vi "FILE_DIALOG 2016.vi"(0 "flow_slope_IN":dbl=51.35 format="%.2f", 1 "pressure_slope_IN":dbl=23.33 format="%.2f", 3 "string_pot_slope_IN":dbl=1.5 format="%.2f", 4 "Descriptions":string[](array[string]), 5 "error in (no error)":errorcluster, 6 "start path":path=path "D:/Cascade/Data/Output Files", 7 "Sensor Cluster":T1, 10 "Array in":refnum<k24>[](array[refnum])) -> (8 "path":path, 9 "Sensor Cluster 2":T1, 11 "exists":bool, 12 "Array out":refnum<k24>[](array[refnum]), 14 "flow_slope_OUT":dbl=51.35 format="%.2f", 15 "pressure_slope_OUT":dbl=732.5347533511234 format="%.2f", 17 "string_pot_slope_OUT":dbl=1.5 format="%.2f", 19 "error out":errorcluster)   [LabVIEW 2016]
uses:
  C:/Program Files (x86)/National Instruments/LabVIEW 2016/vi.lib/ULx/ULx_LV.dll
  Program Files (x86)/National Instruments/LabVIEW 2016/vi.lib/ULx/ULx_LV.dll
  controls/MCC DAQ Readings.ctl
panel:
  out "Loop Counter":i32
  out "cal_completed":bool
  out "new_or _prev_file_selected":bool
  in  "calibrate_KPRO":bool
  in  "previous_file":bool
  in  "new_file":bool
  in  "OK Button":bool
  # "Select root file\nsuch as test.csv"
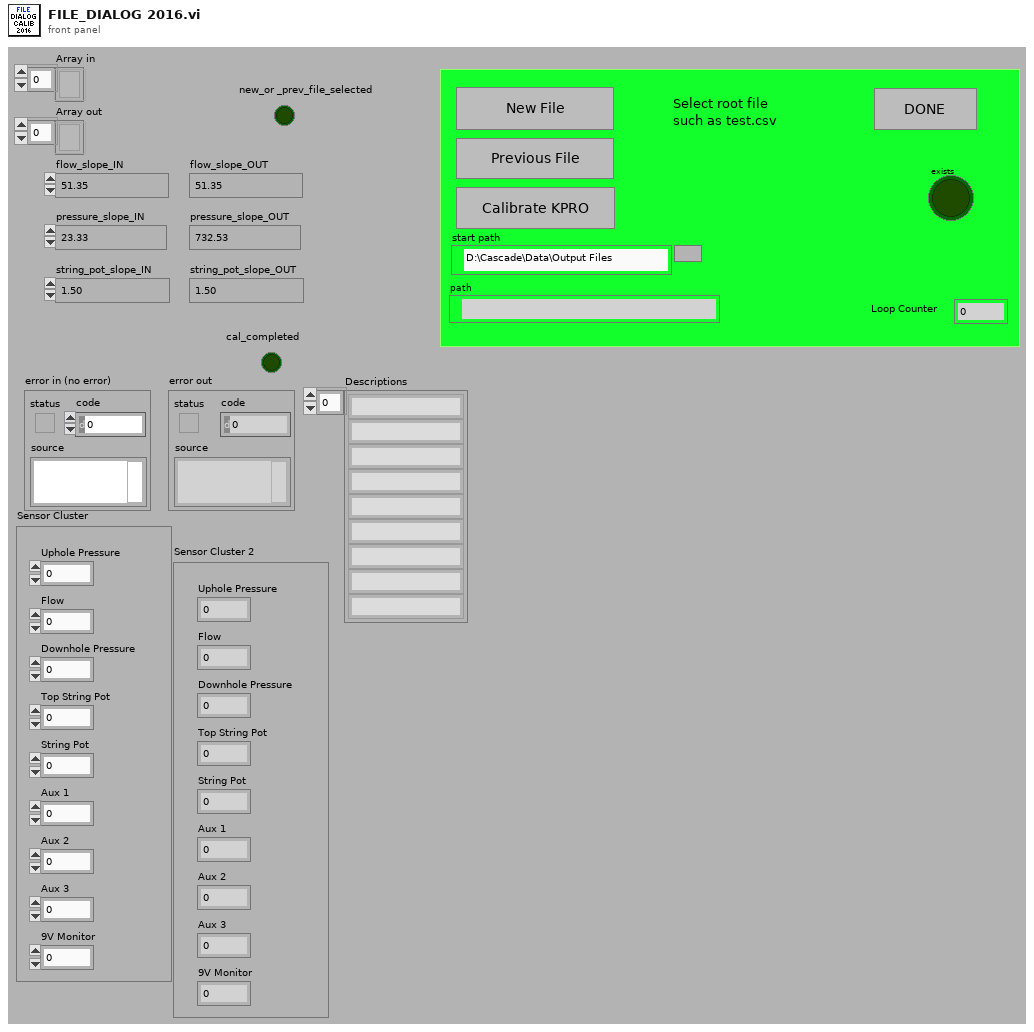
[diagram p1: front panel]
types:
  T1 = typedef "MCC DAQ Readings.ctl" = cluster{"Uphole Pressure":dbl, "Flow":dbl, "Downhole Pressure":dbl, "Top String Pot":dbl, "String Pot":dbl, "Aux 1":dbl, "Aux 2":dbl, "Aux 3":dbl, "9V Monitor":dbl}
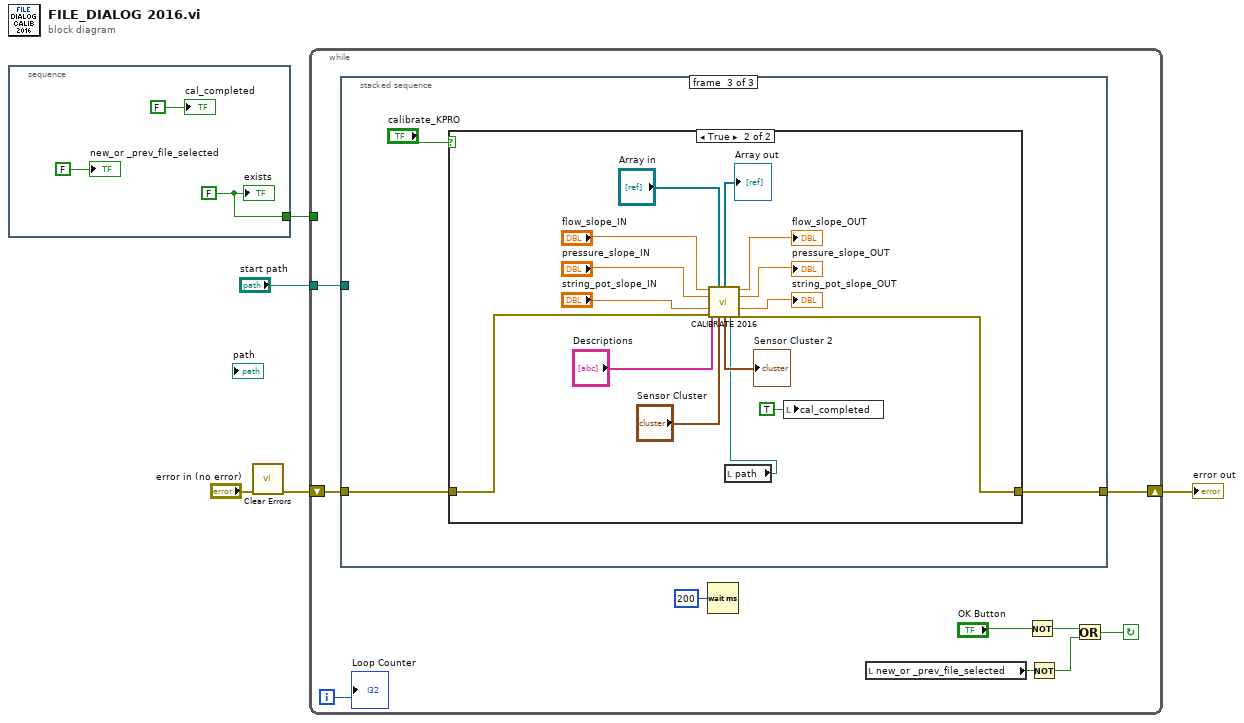
[diagram p0: block diagram]
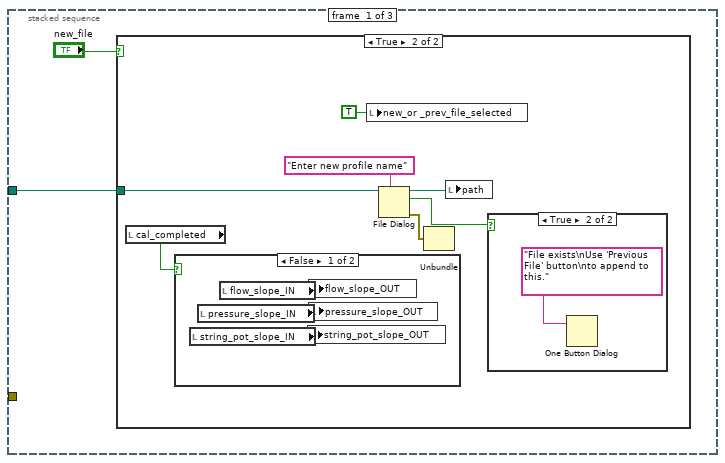
[diagram p2: hidden frame]
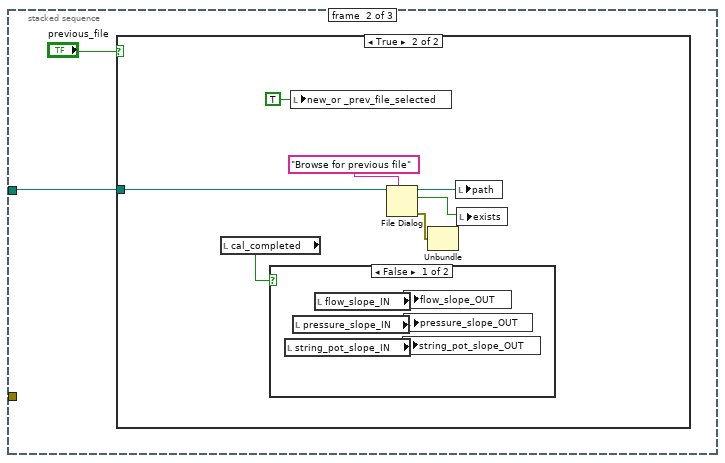
[diagram p6: hidden frame]
diagram:
  n1 = stacked-sequence {
    tunnel: [w8] -> w5
    frame #0 {
      w8 = FALSE ("exists")
      "exists" <- w8
      "new_or _prev_file_selected" <- FALSE ("new_or _prev_file_selected")
      "cal_completed" <- FALSE ("cal_completed")
    }
  }
  n2 = call <vilib>:"Clear Errors.vi"("error in (no error)"="error in (no error)") -> ("error out"=w1:errorcluster)  [unwired: 5 in, 1 out]
  n3 = while {
    shift-left: w1 -> [w15]
    shift-right: [w14] -> w2
    tunnel: "start path" -> [w16]
    tunnel: w5 -> [_]
    i -> [w9]
    stop <- w13 continue-if-true
    n4 = stacked-sequence {
      tunnel: w16 -> [w19 w32 _]
      tunnel: w15 -> [_ _ w45]
      tunnel: [_ _ w44] -> w14
      frame #0 {
        n5 = case shown="True" "new_file" {
          tunnel: w19 -> [_ w24]
          frame False {
          }
          frame True {
            n6 = local read "cal_completed"() -> (w22:bool)
            n7 = case shown="False" w22 {
              frame False {
                n8 = local read "string_pot_slope_IN"() -> (w28:dbl)
                n9 = local read "pressure_slope_IN"() -> (w29:dbl)
                n10 = local read "flow_slope_IN"() -> (w30:dbl)
                n11 = local write "string_pot_slope_OUT"(w28) -> ()
                n12 = local write "flow_slope_OUT"(w30) -> ()
                n13 = local write "pressure_slope_OUT"(w29) -> ()
              }
              frame True {
              }
            }
            n14 = local write "new_or _prev_file_selected"(TRUE ("new_or _prev_file_selected")) -> ()
            n15 = File Dialog(7:"Enter new profile name" ("prompt"), 11:w24) -> (0:w21:errorcluster, 2:w25:bool, 3:w26:path)  [unwired: 5 in, 1 out]
            n16 = Unbundle(w21) -> ()  [unwired: 3 out]
            n17 = local write "path"(w26) -> ()
            n18 = case shown="True" w25 {
              frame False {
              }
              frame True {
                n19 = One Button Dialog(message="File exists\nUse 'Previous File' button\nto append to this.") -> ()  [unwired: 1 in, 1 out]
              }
            }
          }
        }
      }
      frame #1 {
        n20 = case shown="True" "previous_file" {
          tunnel: w32 -> [_ w37]
          frame False {
          }
          frame True {
            n21 = local read "cal_completed"() -> (w35:bool)
            n22 = case shown="False" w35 {
              frame False {
                n23 = local read "string_pot_slope_IN"() -> (w41:dbl)
                n24 = local read "pressure_slope_IN"() -> (w42:dbl)
                n25 = local read "flow_slope_IN"() -> (w43:dbl)
                n26 = local write "string_pot_slope_OUT"(w41) -> ()
                n27 = local write "flow_slope_OUT"(w43) -> ()
                n28 = local write "pressure_slope_OUT"(w42) -> ()
              }
              frame True {
              }
            }
            n29 = local write "new_or _prev_file_selected"(TRUE ("new_or _prev_file_selected")) -> ()
            n30 = File Dialog(7:"Browse for previous file" ("prompt"), 11:w37) -> (0:w34:errorcluster, 2:w38:bool, 3:w39:path)  [unwired: 5 in, 1 out]
            n31 = Unbundle(w34) -> ()  [unwired: 3 out]
            n32 = local write "path"(w39) -> ()
            n33 = local write "exists"(w38) -> ()
          }
        }
      }
      frame #2 {
        n34 = case shown="True" "calibrate_KPRO" {
          tunnel: w45 -> [w47 w59]
          tunnel: [w47 w58] -> w44
          frame False {
          }
          frame True {
            n35 = local read "path"() -> (w48:path)
            n36 = call "CALIBRATE 2016.vi"("flow_slope_IN"="flow_slope_IN", "Array in"="Array in", "pressure_slope_IN"="pressure_slope_IN", "Descriptions"="Descriptions", "string_pot_slope_IN"="string_pot_slope_IN", "error in (no error)"=w59, "Sensor Cluster"="Sensor Cluster", "Path"=w48) -> ("Array out"=→"Array out":refnum<k24>[], "flow_slope_OUT"=→"flow_slope_OUT":dbl, "pressure_slope_OUT"=→"pressure_slope_OUT":dbl, "string_pot_slope_OUT"=→"string_pot_slope_OUT":dbl, "Sensor Cluster 2"=→"Sensor Cluster 2":T1, "error out"=w58:errorcluster)  [unwired: 2 in]
            n37 = local write "cal_completed"(TRUE ("cal_completed")) -> ()
          }
        }
      }
    }
    n38 = Wait (ms)(milliseconds to wait=u32 200) -> ()  [unwired: 1 out]
    n39 = local read "new_or _prev_file_selected"() -> (w11:bool)
    n40 = Not(x="OK Button") -> (.not. x?=w12:bool)
    n41 = Not(x=w11) -> (.not. x?=w10:bool)
    n42 = Or(x=w12, y=w10) -> (x .or. y?=w13:bool)
    "Loop Counter" <- w9
  }
  "error out" <- w2
